vi "Embedded TDMS Logger.Async.vi"(10 "Parameters":variant, 11 "Process":refnum<class "Process.lvclass">) -> ()   [LabVIEW 2023, in "Embedded TDMS Logger Engine.lvlib"]
uses:
  Embedded TDMS Logger Engine.lvlib
  <vilib>/NI/NIVS Inline Async API/_VS Inline Async API/Process/Process.lvclass
  <vilib>/NI/NIVS Inline Async API/_VS Inline Async API/Process/Process.lvclass/Process.ctl
  Shared/Compiled.Settings.ctl
  Shared/FileData.ctl
  Shared/GroupData.ctl
  Shared/Meta Data Item.ctl
  Shared/ChannelData.ctl
  <vilib>/NI VeriStand/Custom Device API/Data Reference.ctl
  Shared/SegmentOptions.ctl
  <vilib>/NI/NIVS Inline Async API/_Data Access Engine/Access Type Classes/Read/Read.lvclass/Read.ctl
  <vilib>/NI/NIVS Inline Async API/_Data Access Engine/Data Access Engine/Methods/Read.Data.vi
  <vilib>/NI/NIVS Inline Async API/_VS Inline Async API/Process/Data Member Access/Read Data Access.vi
  <vilib>/NI/NIVS Inline Async API/_VS Inline Async API/Error Handling Process/SubVIs/Error.ConvertArray.vi
  <vilib>/NI/NIVS Inline Async API/_Data Access Engine/Access Type Classes/Read/Read.ProcessData.vi
  <vilib>/NI/NIVS Inline Async API/_Data Access Engine/Data Access Engine/Methods/Read.Lookup.vi
  <vilib>/NI VeriStand/Custom Device API/Global Data Refs.vi
  <vilib>/NI/NIVS Inline Async API/_Data Access Engine/Data Access Engine/Data Access Engine.lvclass
  Shared/Embedded TDMS Logger Shared.lvlib
  <vilib>/NI VeriStand/Custom Device API/Custom Device API.lvlib
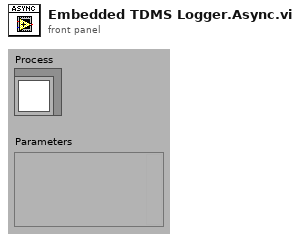
[diagram p1: front panel]
types:
  T1 = typedef "Embedded TDMS Logger Shared.lvlib/Compiled.Settings.ctl" = cluster{"Name":string, "Async Init Timeout":u16, "File Data":T2, "Segment Files":bool, "Segment Every":dbl, "Trigger?":bool, "Segment by":T7, "Trigger Ref":T6}
  T2 = typedef "Embedded TDMS Logger Shared.lvlib/FileData.ctl" = cluster{"Date Captured":string, "Directory":string, "Name":string, "Groups":T3[], "Meta Data":T4[]}
  T3 = typedef "Embedded TDMS Logger Shared.lvlib/GroupData.ctl" = cluster{"Data Rate":string, "Meta Data":T4[], "Channels":T5[], "Name":string}
  T4 = typedef "Embedded TDMS Logger Shared.lvlib/Meta Data Item.ctl" = cluster{"Key":string, "Value":string}
  T5 = typedef "Embedded TDMS Logger Shared.lvlib/ChannelData.ctl" = cluster{"Name":string, "Meta Data":T4[], "Data Reference":T6, "Wfm?":bool, "Increment":dbl}
  T6 = typedef "Custom Device API.lvlib/Data Reference.ctl" = i32
  T7 = typedef "SegmentOptions.ctl" = enum16{"Time (s)", "Size (MB)"}
  T8 = typedef "Data Access Engine.lvlib/Data Access Engine.lvclass/Read.DVR.ctl" = refnum<data-value>
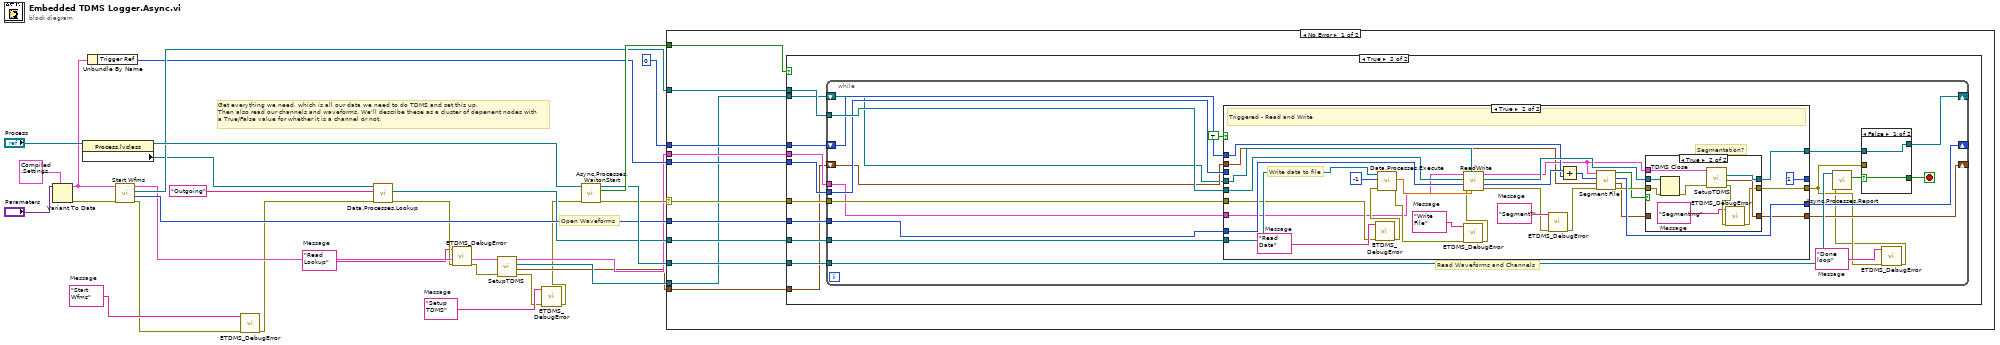
[diagram p0: block diagram]
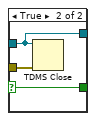
[diagram p3: hidden frame]
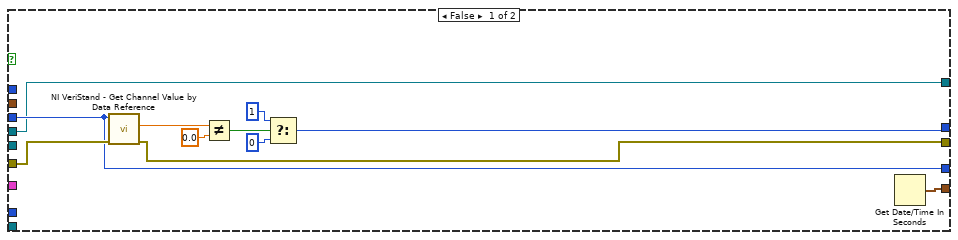
[diagram p4: hidden frame]
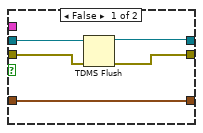
[diagram p5: hidden frame]
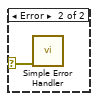
[diagram p6: hidden frame]
diagram:
  w3 = "Setup TDMS"  # Message
  w5 = "Read Lookup"  # Message
  w9 = "Start Wfms"  # Message
  # "Open Waveforms"
  # "Get everything we need, which is all our data we need to do TDMS and set this up.\nThen also read our channels and waveforms. We'll describe these as a cluster of depenent nodes with\na True/False value for whether it is a channel or not."
  n1 = Variant To Data(type=T1 {"Name"="", "Async Init Timeout"=0, "File Data"={"Date Captured"="", "Directory"="", "Name"="", "Groups"=[], "Meta Data"=[]}, "Segment Files"=FALSE, "Segment Every"=0.0, "Trigger?"=FALSE, "Segment by"=enum."Size (MB)", "Trigger Ref"=0} ("Compiled.Settings"), Variant="Parameters") -> (data=w15:T1, error out=w14:errorcluster)  [unwired: 1 in]
  n2 = property class="Process.lvclass"(reference="Process") -> (reference out=w25:refnum<class "Process.lvclass">, "Data Member Access:Data Access"=w16:refnum<class "Data Access Engine.lvclass">)  [unwired: 1 in, 1 out]
  n3 = Unbundle By Name(w15) -> ("Trigger Ref"=w19:T6)
  n4 = call "Start Wfms.vi"("error in (no error)"=w14, "Compiled.Settings"=w15) -> ("error out"=w8:errorcluster, "Channel Refs"=w21:T6[], "Wfm Refs"=w22:refnum<class "Single Waveform Read (DBL).lvclass">[], "Compiled.Settings Out"=w12:T1)  [unwired: 6 in]
  n5 = call "ETDMS_DebugError.vi"("error in (no error)"=w8, "Message"=w9) -> ("error out"=w7:errorcluster)  [unwired: 9 in]
  n6 = call-poly <vilib>:"Data.Processes.Lookup.vi"("error in (no error)"=w7, "Name"="Outgoing", "Data Access API in"=w16) -> ("error out"=w6:errorcluster, "Ref"=w17:T8)  [unwired: 5 in, 2 out]
  n7 = call "ETDMS_DebugError.vi"("error in (no error)"=w6, "Message"=w5) -> ("error out"=w4:errorcluster)  [unwired: 9 in]
  n8 = call "SetupTDMS.vi"("error in (no error)"=w4, "Compiled.Settings In"=w12) -> ("error out"=w2:errorcluster, "File Start Time"=w10:timestamp, "tdms file out"=w13:refnum<k34>, "Compiled.Settings Out"=w11:T1)  [unwired: 6 in]
  n9 = call "ETDMS_DebugError.vi"("error in (no error)"=w2, "Message"=w3) -> ("error out"=w1:errorcluster)  [unwired: 9 in]
  n10 = call <vilib>:"Async.Processes.WaitonStart.vi"("error in (no error)"=w1, "Process"=w25) -> ("error out"=w27:errorcluster, "Execute"=w29:bool, "Process out"=w28:refnum<class "Process.lvclass">)  [unwired: 7 in]
  n11 = case shown="No Error" w27 {
    selector: w27 -> [w38 w131]
    tunnel: w29 -> [w40 _]
    tunnel: w28 -> [w39 _]
    tunnel: w11 -> [w37 _]
    tunnel: w22 -> [w36 _]
    tunnel: w21 -> [w35 _]
    tunnel: u64 0 -> [w34 _]
    tunnel: w19 -> [w33 _]
    tunnel: w17 -> [w32 _]
    tunnel: w13 -> [w31 _]
    tunnel: w10 -> [w30 _]
    frame No Error {
      n12 = case shown="True" w40 {
        tunnel: w38 -> [_ w49]
        tunnel: w39 -> [_ w50]
        tunnel: w37 -> [_ w48]
        tunnel: w36 -> [_ w47]
        tunnel: w35 -> [_ w46]
        tunnel: w34 -> [_ w45]
        tunnel: w33 -> [_ w44]
        tunnel: w32 -> [_ w43]
        tunnel: w31 -> [_ w42]
        tunnel: w30 -> [_ w41]
        frame False {
        }
        frame True {
          n13 = while {
            tunnel: w49 -> [w57]
            tunnel: w50 -> [w70]
            shift-right: [w60] -> _
            shift-left: w42 -> [w55]
            tunnel: w48 -> [w51]
            tunnel: w47 -> [w69]
            tunnel: w46 -> [w68]
            shift-right: [w65] -> _
            shift-left: w45 -> [w67]
            shift-right: [w66] -> _
            shift-left: w41 -> [w56]
            tunnel: w44 -> [w59]
            tunnel: w43 -> [w64]
            stop <- w62 stop-if-true
            w54 = "Done loop"  # Message
            # "Read Waveforms and Channels"
            n14 = case shown="True" TRUE {
              tunnel: [w76 w116] -> w61
              tunnel: [w83 w115] -> w53
              tunnel: w55 -> [w76 w114]
              tunnel: w57 -> [w84 w95]
              tunnel: w69 -> [_ w112]
              tunnel: w68 -> [_ w111]
              tunnel: w67 -> [_ w109]
              tunnel: [w77 w101] -> w66
              tunnel: [w79 w107] -> w65
              tunnel: w56 -> [_ w104]
              tunnel: w59 -> [w79 _]
              tunnel: [w78 1] -> _
              tunnel: w64 -> [_ w98]
              tunnel: w51 -> [_ w87]
              frame False {
                n15 = call <vilib>:"NI VeriStand - Get Channel Value by Data Reference.vi"("error in (no error)"=w84, "Data Reference in"=w79) -> ("error out"=w83:errorcluster, "Value"=w85:dbl)  [unwired: 8 in]
                n16 = Not Equal?(x=w85, y=0.0) -> (x != y?=w82:bool)
                n17 = Select(t=u64 1, s=w82, f=u64 0) -> (s? t:f=w78:u64)
                n18 = Get Date/Time In Seconds() -> (seconds since 1Jan1904=w77:timestamp)
              }
              frame True {
                w90 = "Segment?"  # Message
                w93 = "Write File"  # Message
                w96 = "Read Data"  # Message
                # "Write data to file"
                # "Segmentation?"
                # "Triggered - Read and Write"
                n19 = call "ETDMS_DebugError.vi"("error in (no error)"=w95, "Message"=w96) -> ("error out"=w94:errorcluster)  [unwired: 9 in]
                n20 = call-poly <vilib>:"Data.Processes.Execute.vi"("error in (no error)"=w94, "timeout ms"=-1, "Ref"=w98) -> ("error out"=w92:errorcluster, "Values"=w99:dbl[])  [unwired: 6 in, 1 out]
                n21 = call "ETDMS_DebugError.vi"("error in (no error)"=w92, "Message"=w93) -> ("error out"=w91:errorcluster)  [unwired: 9 in]
                n22 = call "ReadWrite.vi"("Values"=w99, "tdms file in"=w114, "error in (no error)"=w91, "Channel Refs"=w111, "Wfm Refs"=w112, "Compiled.Settings"=w87) -> ("error out"=w89:errorcluster, "Bytes Written"=w110:u64, "tdms file out"=w113:refnum<k34>, "Compiled.Settings Out"=w108:T1)  [unwired: 2 in]
                n23 = call "ETDMS_DebugError.vi"("error in (no error)"=w89, "Message"=w90) -> ("error out"=w88:errorcluster)  [unwired: 9 in]
                n24 = Add(x=w110, y=w109) -> (x+y=w103:u64)
                n25 = call "Segment File.vi"("error in (no error)"=w88, "current time in"=w104, "Current Bytes in"=w103, "Compiled.Settings"=w108) -> ("error out"=w106:errorcluster, "current time out"=w100:timestamp, "Current Bytes out"=w107:u64, "Boolean"=w105:bool)  [unwired: 4 in]
                n26 = case shown="True" w105 {
                  tunnel: w113 -> [w120 w129]
                  tunnel: [w119 w128] -> w116
                  tunnel: [w118 w122] -> w115
                  tunnel: w106 -> [w117 w127]
                  tunnel: w108 -> [_ w126]
                  tunnel: [w121 w125] -> w101
                  tunnel: w100 -> [w121 _]
                  frame False {
                    n27 = TDMS Flush(4:w117, 7:w120) -> (0:w118:errorcluster, 3:w119:refnum<k34>)
                  }
                  frame True {
                    w123 = "Segmenting"  # Message
                    n28 = TDMS Close(8:w127, 11:w129) -> (0:w130:errorcluster)  [unwired: 1 out]
                    n29 = call "SetupTDMS.vi"("error in (no error)"=w130, "Compiled.Settings In"=w126) -> ("error out"=w124:errorcluster, "File Start Time"=w125:timestamp, "tdms file out"=w128:refnum<k34>)  [unwired: 6 in, 1 out]
                    n30 = call "ETDMS_DebugError.vi"("error in (no error)"=w124, "Message"=w123) -> ("error out"=w122:errorcluster)  [unwired: 9 in]
                  }
                }
              }
            }
            n31 = call "ETDMS_DebugError.vi"("error in (no error)"=w53, "Message"=w54) -> ("error out"=w52:errorcluster)  [unwired: 9 in]
            n32 = call <vilib>:"Async.Processes.Report.vi"("Error"=w52, "Process in"=w70) -> ("Stop"=w63:bool)  [unwired: 8 in, 1 out]
            n33 = case shown="False" w63 {
              selector: w63 -> [w72 w75]
              tunnel: [w72 w75] -> w62
              tunnel: w61 -> [w71 w73]
              tunnel: w53 -> [_ w74]
              tunnel: [w71 w73] -> w60
              frame False {
              }
              frame True {
                n34 = TDMS Close(8:w74, 11:w73) -> ()  [unwired: 2 out]
              }
            }
          }
        }
      }
    }
    frame Error {
      n35 = call <vilib>:"Simple Error Handler.vi"("error in (no error)"=w131) -> ()  [unwired: 4 in, 5 out]
    }
  }
